vi "Client.vi"() -> ()   [LabVIEW 2019]
uses:
  Singleton/singleton.lvclass
panel:
  in  "Stop Button":bool
  out "Dummy":bool
  in  "Toggle":bool
  # "The DVR becomes invalid when its\noriginator leaves memory."
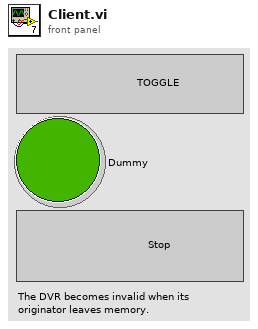
[diagram p1: front panel]
types:
  T1 = typedef "singleton.lvclass/Instance Handle.ctl" = refnum<data-value>
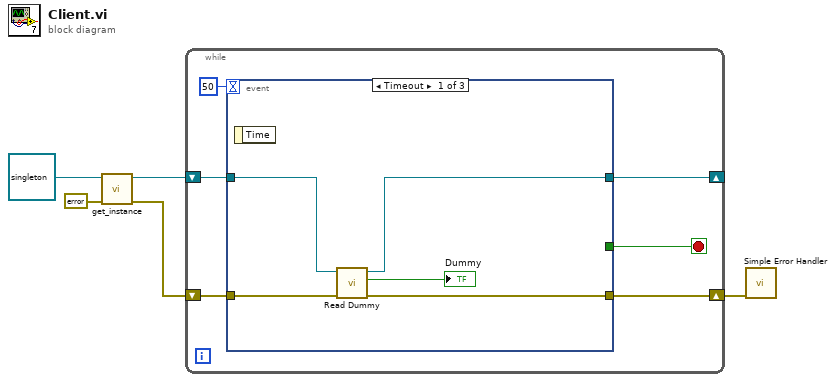
[diagram p0: block diagram]
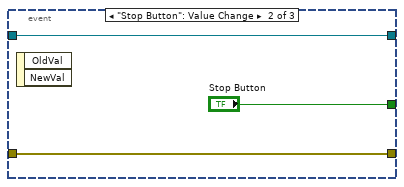
[diagram p2: hidden frame]
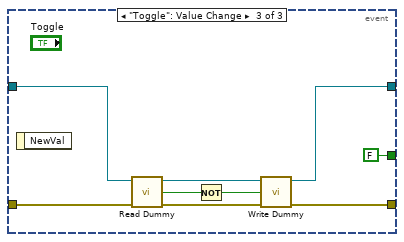
[diagram p3: hidden frame]
diagram:
  n1 = call "get_instance.vi"("error in (no error)"=errorcluster {"status"=FALSE, "code"=0, "source"=""}, "singleton in"=refnum<class "singleton.lvclass"> refnum ("singleton.lvclass")) -> ("error out"=w3:errorcluster, "instance handle"=w2:T1)  [unwired: 8 in]
  n2 = while {
    shift-right: [w9] -> w1
    shift-left: w3 -> [w10]
    shift-right: [w8] -> _
    shift-left: w2 -> [w11]
    stop <- w7 stop-if-true
    n3 = event shown="[0] Timeout" {
      selector: _ -> [_ _ _]
      dyn-events: _ -> [_ _ _]
      timeout: 50 -> [_ _ _]
      tunnel: w11 -> [w16 w19 w28]
      tunnel: w10 -> [w15 w18 w27]
      tunnel: [w14 w18 w25] -> w9
      tunnel: [w13 w19 w24] -> w8
      tunnel: [_ "Stop Button" FALSE ("Stop Button")] -> w7
      event Timeout {
        n4 = event-data() -> ()  [unwired: 1 in, 1 out]
        n5 = call "Read Dummy.vi"("error in (no error)"=w15, "Instance Handle"=w16) -> ("error out"=w14:errorcluster, "Dummy"=→"Dummy":bool, "Session Handle"=w13:T1)  [unwired: 7 in]
      }
      event "Stop Button": Value Change {
        n6 = event-data() -> ()  [unwired: 1 in, 2 out]
      }
      event "Toggle": Value Change {
        n7 = event-data() -> ()  [unwired: 1 in, 1 out]
        n8 = call "Read Dummy.vi"("error in (no error)"=w27, "Instance Handle"=w28) -> ("error out"=w26:errorcluster, "Dummy"=w22:bool, "Session Handle"=w23:T1)  [unwired: 7 in]
        n9 = Not(x=w22) -> (.not. x?=w21:bool)
        n10 = call "Write Dummy.vi"("error in (no error)"=w26, "Dummy"=w21, "Instance Handle"=w23) -> ("error out"=w25:errorcluster, "Session Handle"=w24:T1)  [unwired: 7 in]
      }
    }
  }
  n11 = call <vilib>:"Simple Error Handler.vi"("error in (no error)"=w1) -> ()  [unwired: 4 in, 5 out]
